vi "SUB_RelaySwitch.vi"(1 "error in":errorcluster, 2 "ON_OFF":bool, 3 "DIO":string) -> (0 "error out":errorcluster)   [LabVIEW 2011]
uses:
  <vilib>/DAQmx/write.llb/DAQmx Write (Digital Bool 1Line 1Point).vi
  <vilib>/DAQmx/create/channels.llb/DAQmx Create Channel (DO-Digital Output).vi
  <vilib>/DAQmx/miscellaneous.llb/DAQmx Fill In Error Info.vi
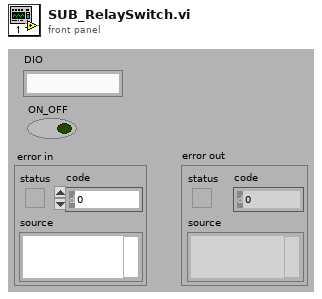
[diagram p1: front panel]
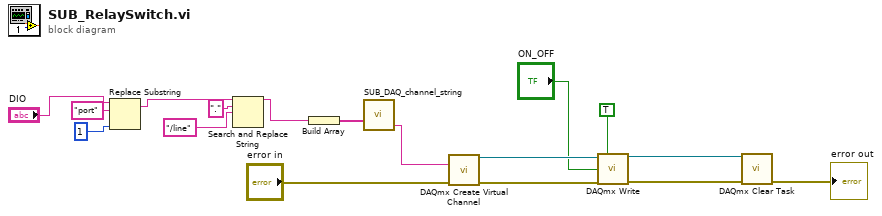
[diagram p0: block diagram]
diagram:
  n1 = Replace Substring(2:1 ("length (len. of substring)"), 4:"port" ("substring (\"\")"), 5:"DIO") -> (1:w8:string)  [unwired: 1 in, 1 out]
  n2 = Search and Replace String(input string=w8, search string=".", replace string="/line" ("replace string (\"\")")) -> (result string=w5:string)  [unwired: 5 in, 3 out]
  n3 = Build Array(w5) -> (w4:string[])
  n4 = call "SUB_DAQ_channel_string.vi"("channel"=w4) -> ("resulting string"=w3:string)  [unwired: 1 in, 2 out]
  n5 = call-poly <vilib>:"DAQmx Create Virtual Channel.vi"("lines"=w3, "error in"="error in") -> ("task out"=w17:refnum<k21>, "error out"=w16:errorcluster)  [unwired: 12 in]
  n6 = call-poly <vilib>:"DAQmx Write.vi"("task/channels in"=w17, "auto start"=TRUE, "data"="ON_OFF", "error in"=w16) -> ("task out"=w14:refnum<k21>, "error out"=w13:errorcluster)  [unwired: 9 in, 1 out]
  n7 = call <vilib>:"DAQmx Clear Task.vi"("task in"=w14, "error in"=w13) -> ("error out"=→"error out":errorcluster)  [unwired: 13 in]
